vi "Access_VersionInfo.vi"(8 "error in":errorcluster, 9 "ModuleVersionInfo":T1, 10 "read/write":enum16{"read", "write"}(ring)) -> (0 "error out":errorcluster, 1 "VersionString":string)   [LabVIEW 2013, in "LVTM.lvlib"]
doc: "reads or writes LV project version information to/from the Windows registry."
uses:
  LVTM.lvlib
  ProductVersion.ctl
  <vilib>/registry/registry.llb/Registry RtKey.ctl
  <vilib>/registry/registry.llb/Read Registry Value Simple STR.vi
  <vilib>/registry/registry.llb/Write Registry Value Simple STR.vi
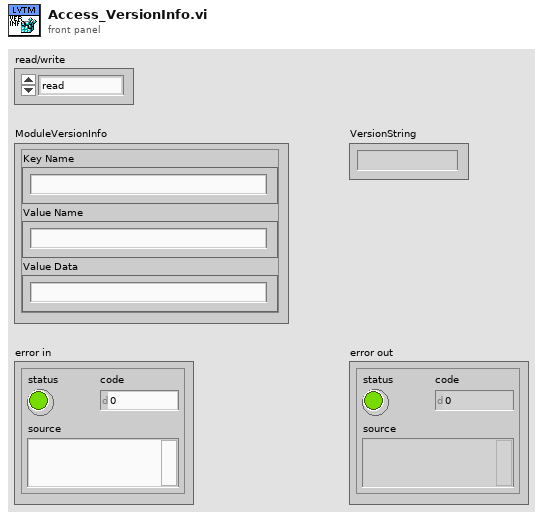
[diagram p1: front panel]
types:
  T1 = typedef "LVTM.lvlib/ProductVersion.ctl" = cluster{"Key Name":string, "Value Name":string, "Value Data":string}
  T2 = typedef "Registry RtKey.ctl" = enum32{"HKEY_CLASSES_ROOT", "HKEY_CURRENT_USER", "HKEY_LOCAL_MACHINE", "HKEY_USERS", "HKEY_PERFORMANCE_DATA", "HKEY_CURRENT_CONFIG", "HKEY_DYN_DATA"}
  T3 = typedef "Registry refnum.ctl" = refnum<k1>
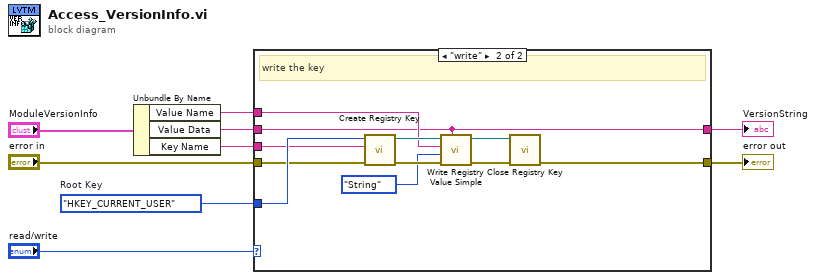
[diagram p0: block diagram]
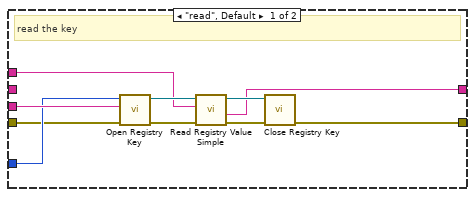
[diagram p2: hidden frame]
diagram:
  w9 = Registry_RtKey."HKEY_CURRENT_USER"  # Root Key
  n1 = Unbundle By Name("ModuleVersionInfo") -> ("Value Name"=w6:string, "Value Data"=w7:string, "Key Name"=w4:string)
  n2 = case shown="\"write\"" "read/write" {
    tunnel: w9 -> [w13 w25]
    tunnel: w7 -> [_ w22]
    tunnel: w6 -> [w15 w24]
    tunnel: w4 -> [w14 w23]
    tunnel: [w12 w22] -> w3
    tunnel: [w11 w20] -> w2
    tunnel: "error in" -> [w10 w21]
    frame "read", Default {
      # "read the key"
      n3 = call <vilib>:"Open Registry Key.vi"("error in (no error)"=w10, "subkey"=w14, "root key (HKEY_LOCAL_MACHINE)"=w13) -> ("error out"=w19:errorcluster, "refnum out"=w18:T3)  [unwired: 7 in]
      n4 = call-poly <vilib>:"Read Registry Value Simple.vi"("error in (no error)"=w19, "value"=w15, "refnum"=w18) -> ("error out"=w16:errorcluster, "String/Binary data"=w12:string, "refnum out"=w17:T3)  [unwired: 3 in, 1 out]
      n5 = call <vilib>:"Close Registry Key.vi"("error in (no error)"=w16, "refnum"=w17) -> ("error out"=w11:errorcluster)  [unwired: 5 in]
    }
    frame "write" {
      # "write the key"
      n6 = call <vilib>:"Create Registry Key.vi"("error in (no error)"=w21, "subkey"=w23, "root key (HKEY_LOCAL_MACHINE)"=w25) -> ("error out"=w28:errorcluster, "refnum out"=w26:T3)  [unwired: 6 in, 1 out]
      n7 = call-poly <vilib>:"Write Registry Value Simple.vi"("String/Binary data"=w22, "error in (no error)"=w28, "simple data type"=enum16{"String", "Binary", "DWORD"}."String", "value"=w24, "refnum"=w26) -> ("error out"=w30:errorcluster, "refnum out"=w29:T3)  [unwired: 3 in]
      n8 = call <vilib>:"Close Registry Key.vi"("error in (no error)"=w30, "refnum"=w29) -> ("error out"=w20:errorcluster)  [unwired: 5 in]
    }
  }
  "VersionString" <- w3
  "error out" <- w2
